vi "Reverse 2D Array Example 01.vi"() -> ()   [LabVIEW 2009]
uses:
  library/Reverse 2D Array/Reverse 2D Array (Boolean).vi
panel:
  out "Array Reversed by Columns":bool[][](array[boolean])
  out "Array Reversed by Rows":bool[][](array[boolean])
  in  "Array":bool[][](array[boolean])=[[TRUE, FALSE, FALSE, FALSE, TRUE, FALSE], [FALSE, FALSE, TRUE, FALSE, FALSE, FALSE], [TRUE, FALSE, FALSE, FALSE, TRUE, TRUE], [FALSE, TRUE, FALSE, TRUE, FALSE, FALSE]]
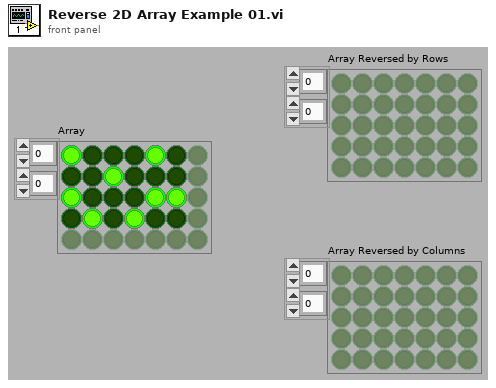
[diagram p1: front panel]
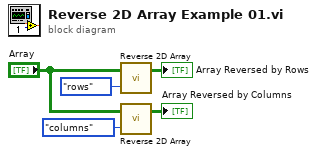
[diagram p0: block diagram]
diagram:
  n1 = call-poly "Reverse 2D Array.vi"("by rows or columns (rows)"=enum16{"rows", "columns"}."rows", "Array"="Array") -> ("Reversed Array"=→"Array Reversed by Rows":bool[][])  [unwired: 1 in]
  n2 = call-poly "Reverse 2D Array.vi"("by rows or columns (rows)"=enum16{"rows", "columns"}."columns", "Array"="Array") -> ("Reversed Array"=→"Array Reversed by Columns":bool[][])  [unwired: 1 in]
